vi "SCT Prepare Initial Variable.vi"(7 "network variables only":bool, 8 "error in (no error)":errorcluster, 9 "new variable?":bool, 10 "default types":T4, 11 "variable in":T5) -> (0 "error out":errorcluster, 1 "Cancelled?":bool, 3 "Variables Out":T1[](array[typedef]))   [LabVIEW 2016]
uses:
  <vilib>/variable/variable.ctl
  <vilib>/variable/Type Descriptor.ctl
  <vilib>/variable/Attribs.ctl
  <resource>/dialog/variable/SCT Default Types.ctl
  <resource>/dialog/variable/SCT Variable.ctl
  <vilib>/variable/NI_Variable.lvlib
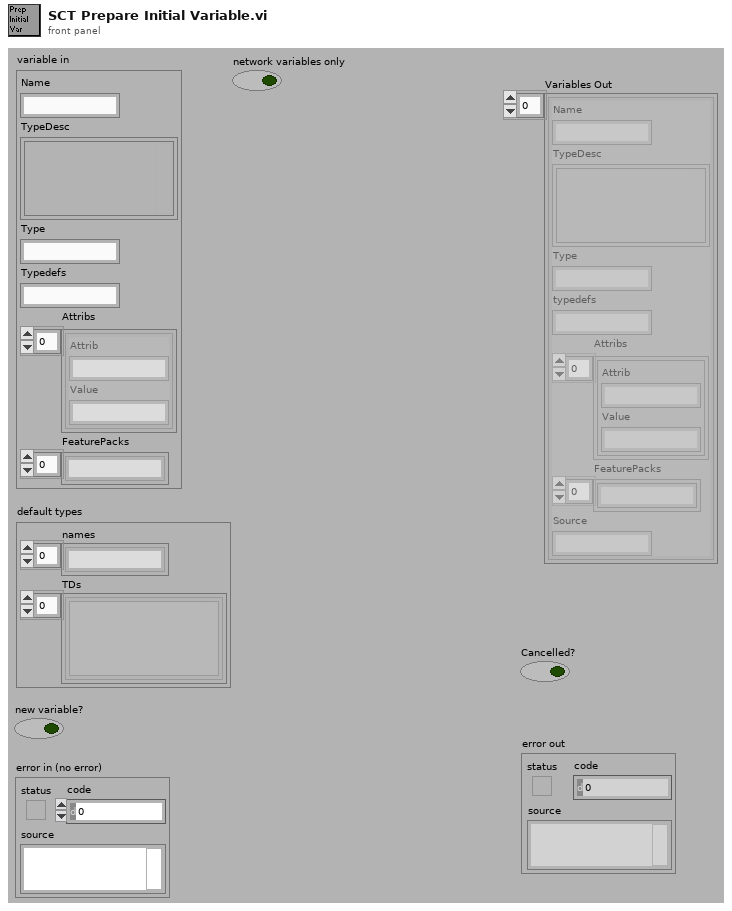
[diagram p1: front panel]
types:
  T1 = typedef "SCT Variable.ctl" = cluster{"Name":string, "TypeDesc":T2, "Type":string, "typedefs":string, "Attribs":T3, "FeaturePacks":string[], "Source":string}
  T2 = typedef "NI_Variable.lvlib/Type Descriptor.ctl" = cluster{"Variant":variant}
  T3 = typedef "NI_Variable.lvlib/Attribs.ctl" = cluster{"Attrib":string, "Value":string}[]
  T4 = typedef "SCT Default Types.ctl" = cluster{"names":string[], "TDs":T2[]}
  T5 = typedef "NI_Variable.lvlib/variable.ctl" = cluster{"Name":string, "TypeDesc":T2, "Type":string, "Typedefs":string, "Attribs":T3, "FeaturePacks":string[]}
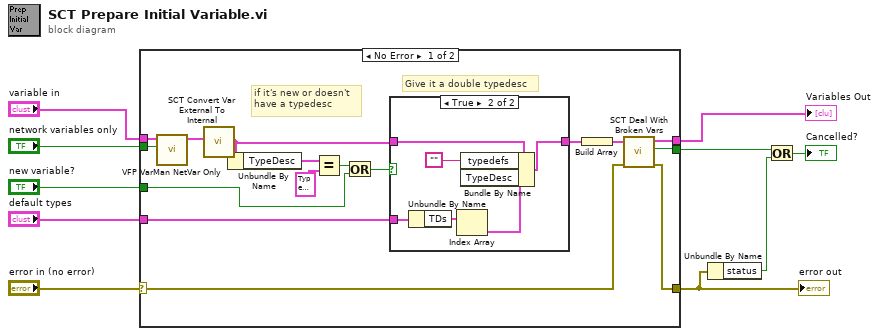
[diagram p0: block diagram]
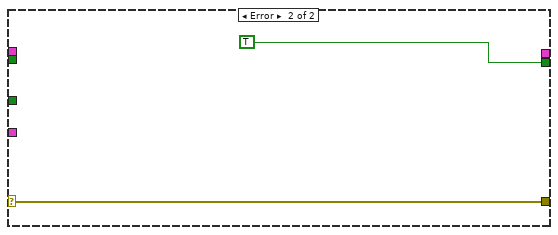
[diagram p3: hidden frame]
diagram:
  n1 = case shown="No Error" "error in (no error)" {
    selector: "error in (no error)" -> [w23 w35]
    tunnel: "variable in" -> [w25 _]
    tunnel: "network variables only" -> [w26 _]
    tunnel: "new variable?" -> [w11 _]
    tunnel: [w24 TRUE ("Cancelled?")] -> w7
    tunnel: "default types" -> [w19 _]
    tunnel: [w22 w35] -> w2
    tunnel: [w21 _] -> w4
    frame No Error {
      # "if it's new or doesn't\nhave a typedesc"
      # "Give it a double typedesc"
      n2 = call <resource>:"VFP VarMan NetVar Only.vi"("Network Variables Only"=w26, "variable in"=w25) -> ("variable out"=w18:T5)  [unwired: 9 in]
      n3 = call <resource>:"SCT Convert Var External To Internal.vi"("External Var"=w18) -> ("Internal Var"=w14:T1)  [unwired: 5 in]
      n4 = Unbundle By Name(w14) -> ("TypeDesc"=w17:T2)
      n5 = Equal?(x=w17, y=T2 {"Variant"=variant} ("TypeDesc")) -> (x = y?=w12:bool)
      n6 = Or(x=w12, y=w11) -> (x .or. y?=w13:bool)
      n7 = case shown="True" w13 {
        tunnel: [w27 w30] -> w15
        tunnel: w14 -> [w27 w31]
        tunnel: w19 -> [_ w29]
        frame False {
        }
        frame True {
          n8 = Unbundle By Name(w29) -> ("TDs"=w33:T2[])
          n9 = Index Array(array=w33) -> (element=w32:T2)  [unwired: 1 in]
          n10 = Bundle By Name(cluster=w31, "typedefs"="", "TypeDesc"=w32) -> (w30:T1)
        }
      }
      n11 = Build Array(w15) -> (w20:T1[])
      n12 = call <resource>:"SCT Deal With Broken Vars.vi"("error in (no error)"=w23, "vars"=w20) -> ("error out"=w22:errorcluster, "Cancelled?"=w24:bool, "vars out"=w21:T1[])  [unwired: 6 in, 1 out]
    }
    frame Error {
    }
  }
  "error out" <- w2
  "Variables Out" <- w4
  n13 = Unbundle By Name(w2) -> ("status"=w1:bool)
  n14 = Or(x=w7, y=w1) -> (x .or. y?=→"Cancelled?":bool)
